vi "init.vi"(8 "error in (no error)":errorcluster, 11 "ESP301_via_TCPIP in":refnum<class "ESP301_via_TCPIP.lvclass">) -> (0 "error out":errorcluster, 3 "ESP301_via_TCPIP out":refnum<class "ESP301_via_TCPIP.lvclass">)   [LabVIEW 2019, in "ESP301_via_TCPIP.lvclass"]
uses:
  ESP301_via_TCPIP.lvclass
  _delayStageBase/_delayStageBase.lvclass
panel:
  in  "max pos":dbl=290.0
  in  "resource name":string
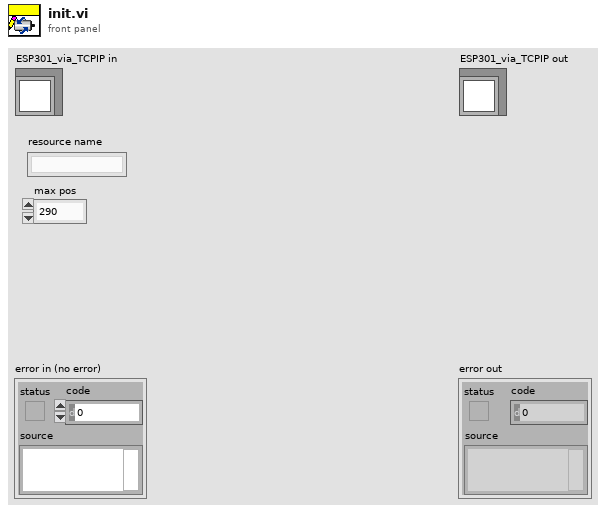
[diagram p1: front panel]
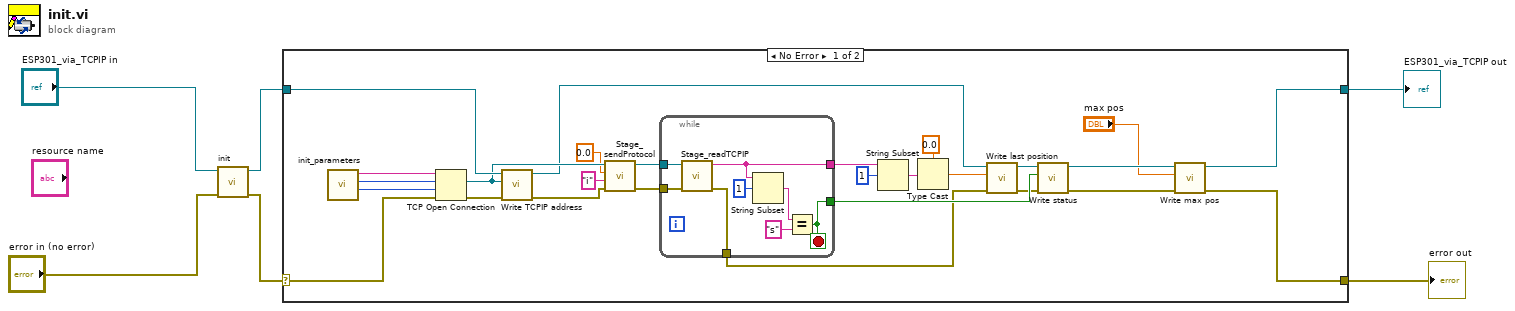
[diagram p0: block diagram]
diagram:
  n1 = call-parent "init.vi"("error in (no error)"="error in (no error)", "_delayStageBase in"="ESP301_via_TCPIP in") -> ("error out"=w1:errorcluster, "_delayStageBase out"=w4:refnum<class "ESP301_via_TCPIP.lvclass">)  [unwired: 8 in]
  n2 = case shown="No Error" w1 {
    selector: w1 -> [w13 w42]
    tunnel: w4 -> [w30 w43]
    tunnel: [w10 w43] -> w3
    tunnel: [w8 w42] -> w2
    frame No Error {
      n3 = call "init_parameters.vi"() -> ("Timeout out"=w32:i32, "Remote port out"=w31:u16, "TCP IP out"=w33:string)  [unwired: 9 in]
      n4 = TCP Open Connection(address=w33, remote port or service name=w31, timeout ms (60000)=w32, error in (no error)=w13) -> (connection ID=w29:refnum<k5>, error out=w12:errorcluster)  [unwired: 1 in]
      n5 = call-dynamic "Write TCPIP address.vi"("error in (no error)"=w12, "TCPIP address"=w29, "ESP301_via_TCPIP in"=w30) -> ("error out"=w23:errorcluster, "ESP301_via_TCPIP out"=w18:refnum<class "ESP301_via_TCPIP.lvclass">)  [unwired: 7 in]
      n6 = call "Stage_sendProtocol.vi"("error in (no error)"=w23, "command"="i", "GoTo position"=0.0, "TCP Network Connection in"=w29) -> ("error out"=w25:errorcluster, "TCP Network Connection out"=w26:refnum<k5>)  [unwired: 6 in]
      n7 = while {
        tunnel: w26 -> [w41]
        tunnel: w25 -> [w40]
        tunnel: [w38] -> w24
        tunnel: [w37] -> w16
        tunnel: [w36] -> w22
        stop <- w38 stop-if-true
        n8 = call "Stage_readTCPIP.vi"("error in (no error)"=w40, "TCP Network Connection in"=w41) -> ("error out"=w37:errorcluster, "data out"=w36:string)  [unwired: 8 in]
        n9 = String Subset(string=w36, length (rest)=1 ("length (rest)")) -> (substring=w34:string)  [unwired: 1 in]
        n10 = Equal?(x=w34, y="s") -> (x = y?=w38:bool)
      }
      n11 = String Subset(string=w22, offset (0)=1) -> (substring=w21:string)  [unwired: 1 in]
      n12 = Type Cast(type=0.0, x=w21) -> (*(type *) &x=w14:dbl)
      n13 = call-dynamic "Write last position.vi"("error in (no error)"=w16, "last position"=w14, "_delayStageBase in"=w18) -> ("error out"=w15:errorcluster, "_delayStageBase out"=w17:refnum<class "ESP301_via_TCPIP.lvclass">)  [unwired: 7 in]
      n14 = call-dynamic "Write status.vi"("error in (no error)"=w15, "status"=w24, "_delayStageBase in"=w17) -> ("error out"=w9:errorcluster, "_delayStageBase out"=w11:refnum<class "ESP301_via_TCPIP.lvclass">)  [unwired: 7 in]
      n15 = call-dynamic "Write max pos.vi"("error in (no error)"=w9, "max pos"="max pos", "_delayStageBase in"=w11) -> ("error out"=w8:errorcluster, "_delayStageBase out"=w10:refnum<class "ESP301_via_TCPIP.lvclass">)  [unwired: 7 in]
    }
    frame Error {
    }
  }
  "error out" <- w2
  "ESP301_via_TCPIP out" <- w3
